vi "Periodic Tasks.vi"(8 "error in":errorcluster) -> ()   [LabVIEW 2015]
doc: "This VI runs in parallel to other tasks. It can contain as many user-defined periodic loops as you need. These can carry out PID or other sorts of timed response."
uses:
  <vilib>/Rock Robotics/WPI/CAN/TalonSRX/WPI_CANTalonSRX_APIControlMode.ctl
  Robot Global Data.vi
  <vilib>/Rock Robotics/WPI/Ultrasonic/WPI_SonarMB1010DigitalRefNum Registry Get.vi
  <vilib>/Rock Robotics/WPI/Ultrasonic/WPI_SonarMB1010DigitalGetRange.vi
  <vilib>/Rock Robotics/Network Tables/NT Write Number.vi
  <vilib>/Rock Robotics/Network Tables/NT Read Number.vi
  <vilib>/addons/control/pid/pid.llb/PID (DBL).vi
  navx-mxp/labview/navX Library v2/navX Library v2.lvlib
  <vilib>/addons/control/pid/NI_PID_pid.lvlib
panel:
  out "Motor Output 2":dbl(graph)
  in  "Intake delay":u32
  in  "Accuracy (+/-)":dbl=0.001 format="%#_13g"
  out "Sensor Velocity":dbl
  out "Distance 2":dbl
  in  "Ramp Rate 2":dbl
  in  "P 2":dbl=0.04
  in  "I 2":dbl=0.000122
  in  "D 2":dbl=0.7
  in  "F 2":dbl=0.0096
  in  "I Zone 2":dbl
  in  "Post beam break delay":u32=200
  in  "Ramp Rate":dbl
  in  "I Zone":dbl
  in  "F":dbl=0.0088
  in  "D":dbl
  in  "I":dbl
  in  "P":dbl
  in  "PID gains Lvl 3":T1={"proportional gain (Kc)"=2.0, "integral time (Ti, min)"=0.0, "derivative time (Td, min)"=0.0003}
  out "Pitch":dbl
  in  "PID Gains Lvl 1":T1={"proportional gain (Kc)"=3.0, "integral time (Ti, min)"=0.0, "derivative time (Td, min)"=0.0}
  out "Motor Output":dbl(graph)
  in  "PID Gains lv 2":T1={"proportional gain (Kc)"=9.0, "integral time (Ti, min)"=0.0, "derivative time (Td, min)"=0.0003}
  out "Potentiometer":dbl
  out "Beam Brake Tripped?":bool
  out "Yaw":dbl
  out "Roll":dbl
  in  "Command limit":dbl=0.25
  in  "Yaw Reset":bool
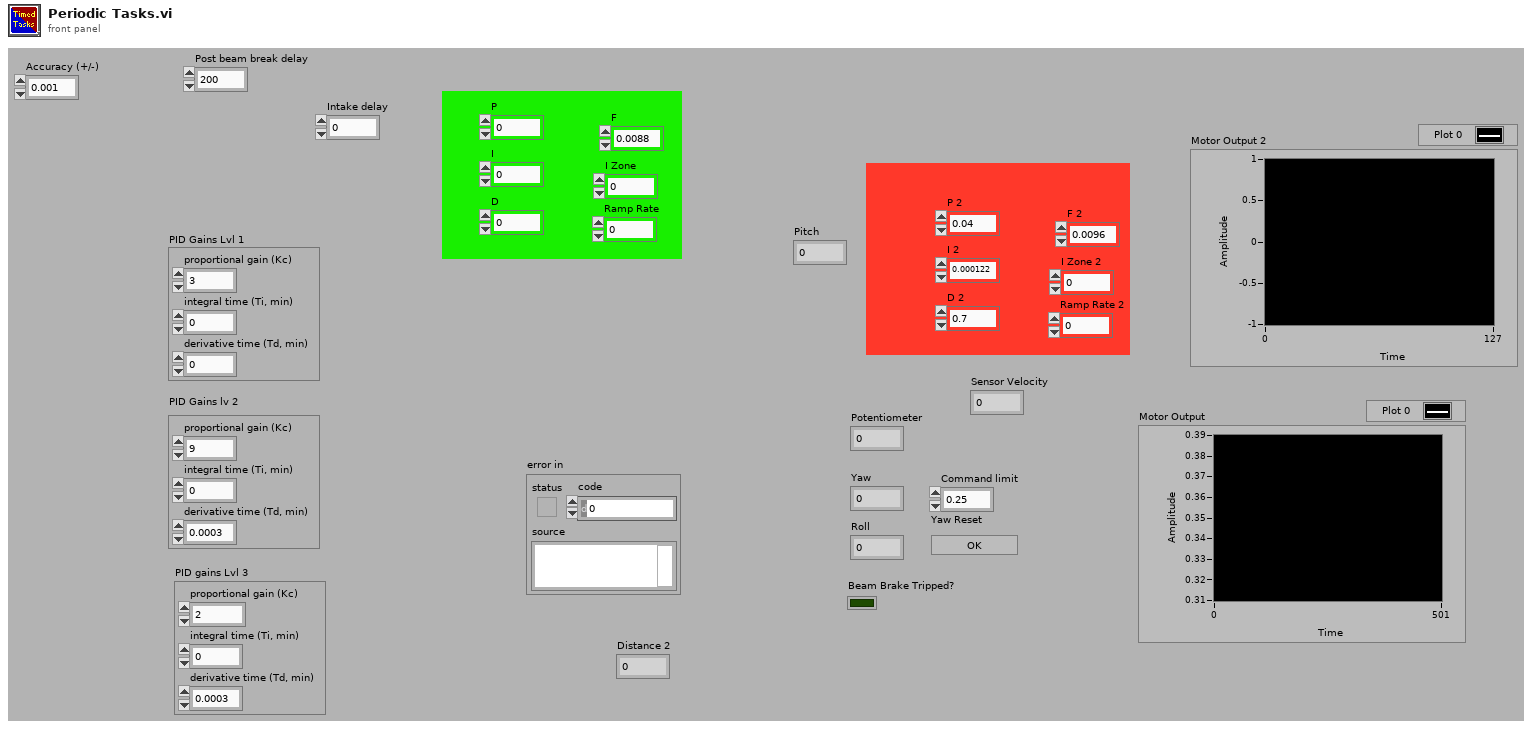
[diagram p1: front panel]
types:
  T1 = cluster{"proportional gain (Kc)":dbl, "integral time (Ti, min)":dbl, "derivative time (Td, min)":dbl}
  T2 = typedef "WPI_SonarMB1010DigitalDeviceRef.ctl" = cluster{"CounterDevRef":T3, "Scaling factor (s/in)":dbl}
  T3 = typedef "WPI_CounterDevRef.ctl" = cluster{"DevStatus":errorcluster, "CntIndex":T4}
  T4 = typedef "FPGA_CounterCtrSystemIndex.ctl" = enum8{"Ctr 0", "Ctr 1", "Ctr 2", "Ctr 3", "Ctr 4", "Ctr 5", "Ctr 6", "Ctr 7", "Invalid"}
  T5 = typedef "navX Library v2.lvlib/Z900_navX_DeviceTypeDef.ctl" = cluster{"Interface":cluster{"Protocol":T6, "Update Rate (4Hz-60Hz)":u8, "navX Open TypeDef":variant}, "Notify Packet":refnum<notifier>, "Loop VI Refnum":refnum<vi>, "Ready to Close Occurrence Refnum":refnum<k4>}
  T6 = typedef "navX Library v2.lvlib/Z900_navX_ProtocolTypeDef.ctl" = enum16{"SERIAL", "I2C", "SPI"}
  T7 = typedef "WPI_PotentiometerDevRef.ctl" = cluster{"DevStatus":errorcluster, "Analog Channel":T8, "Invert Output":bool}
  T8 = typedef "FPGA_AIChannel.ctl" = enum8{"AI 0", "AI 1", "AI 2", "AI 3", "AI MXP 0", "AI MXP 1", "AI MXP 2", "AI MXP 3", "Invalid"}
  T9 = cluster{"Yaw":dbl, "Roll":dbl, "Pitch":dbl, "Heading":dbl, "Fused Heading":dbl}
  T10 = typedef "WPI_DigitalInputDevRef.ctl" = cluster{"DevStatus":errorcluster, "DIO Channel":T11}
  T11 = typedef "FPGA_DIOChannel.ctl" = enum8{"DIO 0", "DIO 1", "DIO 2", "DIO 3", "DIO 4", "DIO 5", "DIO 6", "DIO 7", "DIO 8", "DIO 9", "DIO MXP 0", "DIO MXP 1", "DIO MXP 2", "DIO MXP 3", "DIO MXP 4", "DIO MXP 5", "DIO MXP 6", "DIO MXP 7", "DIO MXP 8", "DIO MXP 9", "DIO MXP 10", "DIO MXP 11", "DIO MXP 12", "DIO MXP 13", "DIO MXP 14", "DIO MXP 15", "Invalid"}
  T12 = typedef "WPI_MotorControlDeviceRef.ctl" = cluster{"DeviceStatus":errorcluster, "Type":T13, "PWM":cluster{"PWM Channel":T14, "DeadBand":T15}, "CAN":cluster{"Device Number":u8, "Control Mode":T16, "Semaphore":T17, "Max Vout":dbl, "TalonSRX Control Mode":T18}, "Invert":bool}
  T13 = typedef "WPI_MotorControlType.ctl" = enum16{"PWM", "CAN", "CANTalonSRX"}
  T14 = typedef "FPGA_DIOPWMChannel.ctl" = enum8{"PWM 0", "PWM 1", "PWM 2", "PWM 3", "PWM 4", "PWM 5", "PWM 6", "PWM 7", "PWM 8", "PWM 9", "PWM MXP 0", "PWM MXP 1", "PWM MXP 2", "PWM MXP 3", "PWM MXP 4", "PWM MXP 5", "PWM MXP 6", "PWM MXP 7", "PWM MXP 8", "PWM MXP 9", "Invalid"}
  T15 = typedef "WPI_PWMDeadband.ctl" = cluster{"Name":string, "maxPositivePwm":i32, "minPositivePwm":i32, "centerPwm":i32, "maxNegativePwm":i32, "minNegativePwm":i32, "angularRange":u16}
  T16 = typedef "WPI_CANJaguar_ControlMode.ctl" = enum8{"Percent VBus", "Current", "Speed", "Position", "Voltage"}
  T17 = typedef "Semaphore RefNum" = refnum<k1>
  T18 = typedef "WPI_CANTalonSRX_APIControlMode.ctl" = enum8{"Percent VBus", "Speed", "Position", "Slave", "Unchanged / Invalid", "Voltage Compensation", "Current", "Motion Profile"}
  T19 = typedef "WPI_CANTalonSRX_GlobalStatus.ctl" = cluster{"Applied Throttle":dbl, "Module Enabled":bool, "CAN Error":errorcluster, "Closed Loop Error":dbl, "Forward Limit Switch Closed":bool, "Reverse Limit Switch Closed":bool, "Sensor Position":dbl, "Sensor Velocity":dbl, "Current":dbl, "Sticky Fault - Over Temp":bool, "Sticky Fault - Under Voltage":bool, "Sticky Fault - Forward Limit":bool, "Sticky Fault - Reverse Limit":bool, "Sticky Fault - Forward Soft Limit":bool, "Sticky Fault - Reverse Soft Limit":bool, "Brake is Enabled":bool, "Encoder Position":dbl, "Encoder Velocity":dbl, "Encoder Index Count":dbl, "Encoder A Pin State":bool, "Encoder B Pin State":bool, "Encoder Index Pin State":bool, "Analog In":dbl, "Analog In Velocity":dbl, "Temperature (C)":dbl, "Battery Voltage":dbl, "Control 5 Is Supported":bool, "Current Profile Slot Select":dbl, "Pos Div 8":bool, "Vel Div 4":bool, "Pulse Width Position":i32, "Pulse Width Velocity":i32, "Pulse Width Rise To Rise (us)":i32, "Pulse Width Rise To Fall (us)":i32, "Mot Prof Active Is Under Run":bool, "Mot Prof Active Has Under Run":bool, "Mot Prof Active Is Last":bool, "Mot Prof Active Velocity Only":bool, "Mot Prof Active Is Valid":bool, "Mot Prof Buffer Is Full":bool, "Mot Prof Active Profile Slot Select":i32, "Mot Prof NextID":i32, "Mot Prof Count":i32, "Mot Prof Active Velocity":dbl, "Mot Prof Active Position":dbl, "Mot Prof Output Enable":i32}
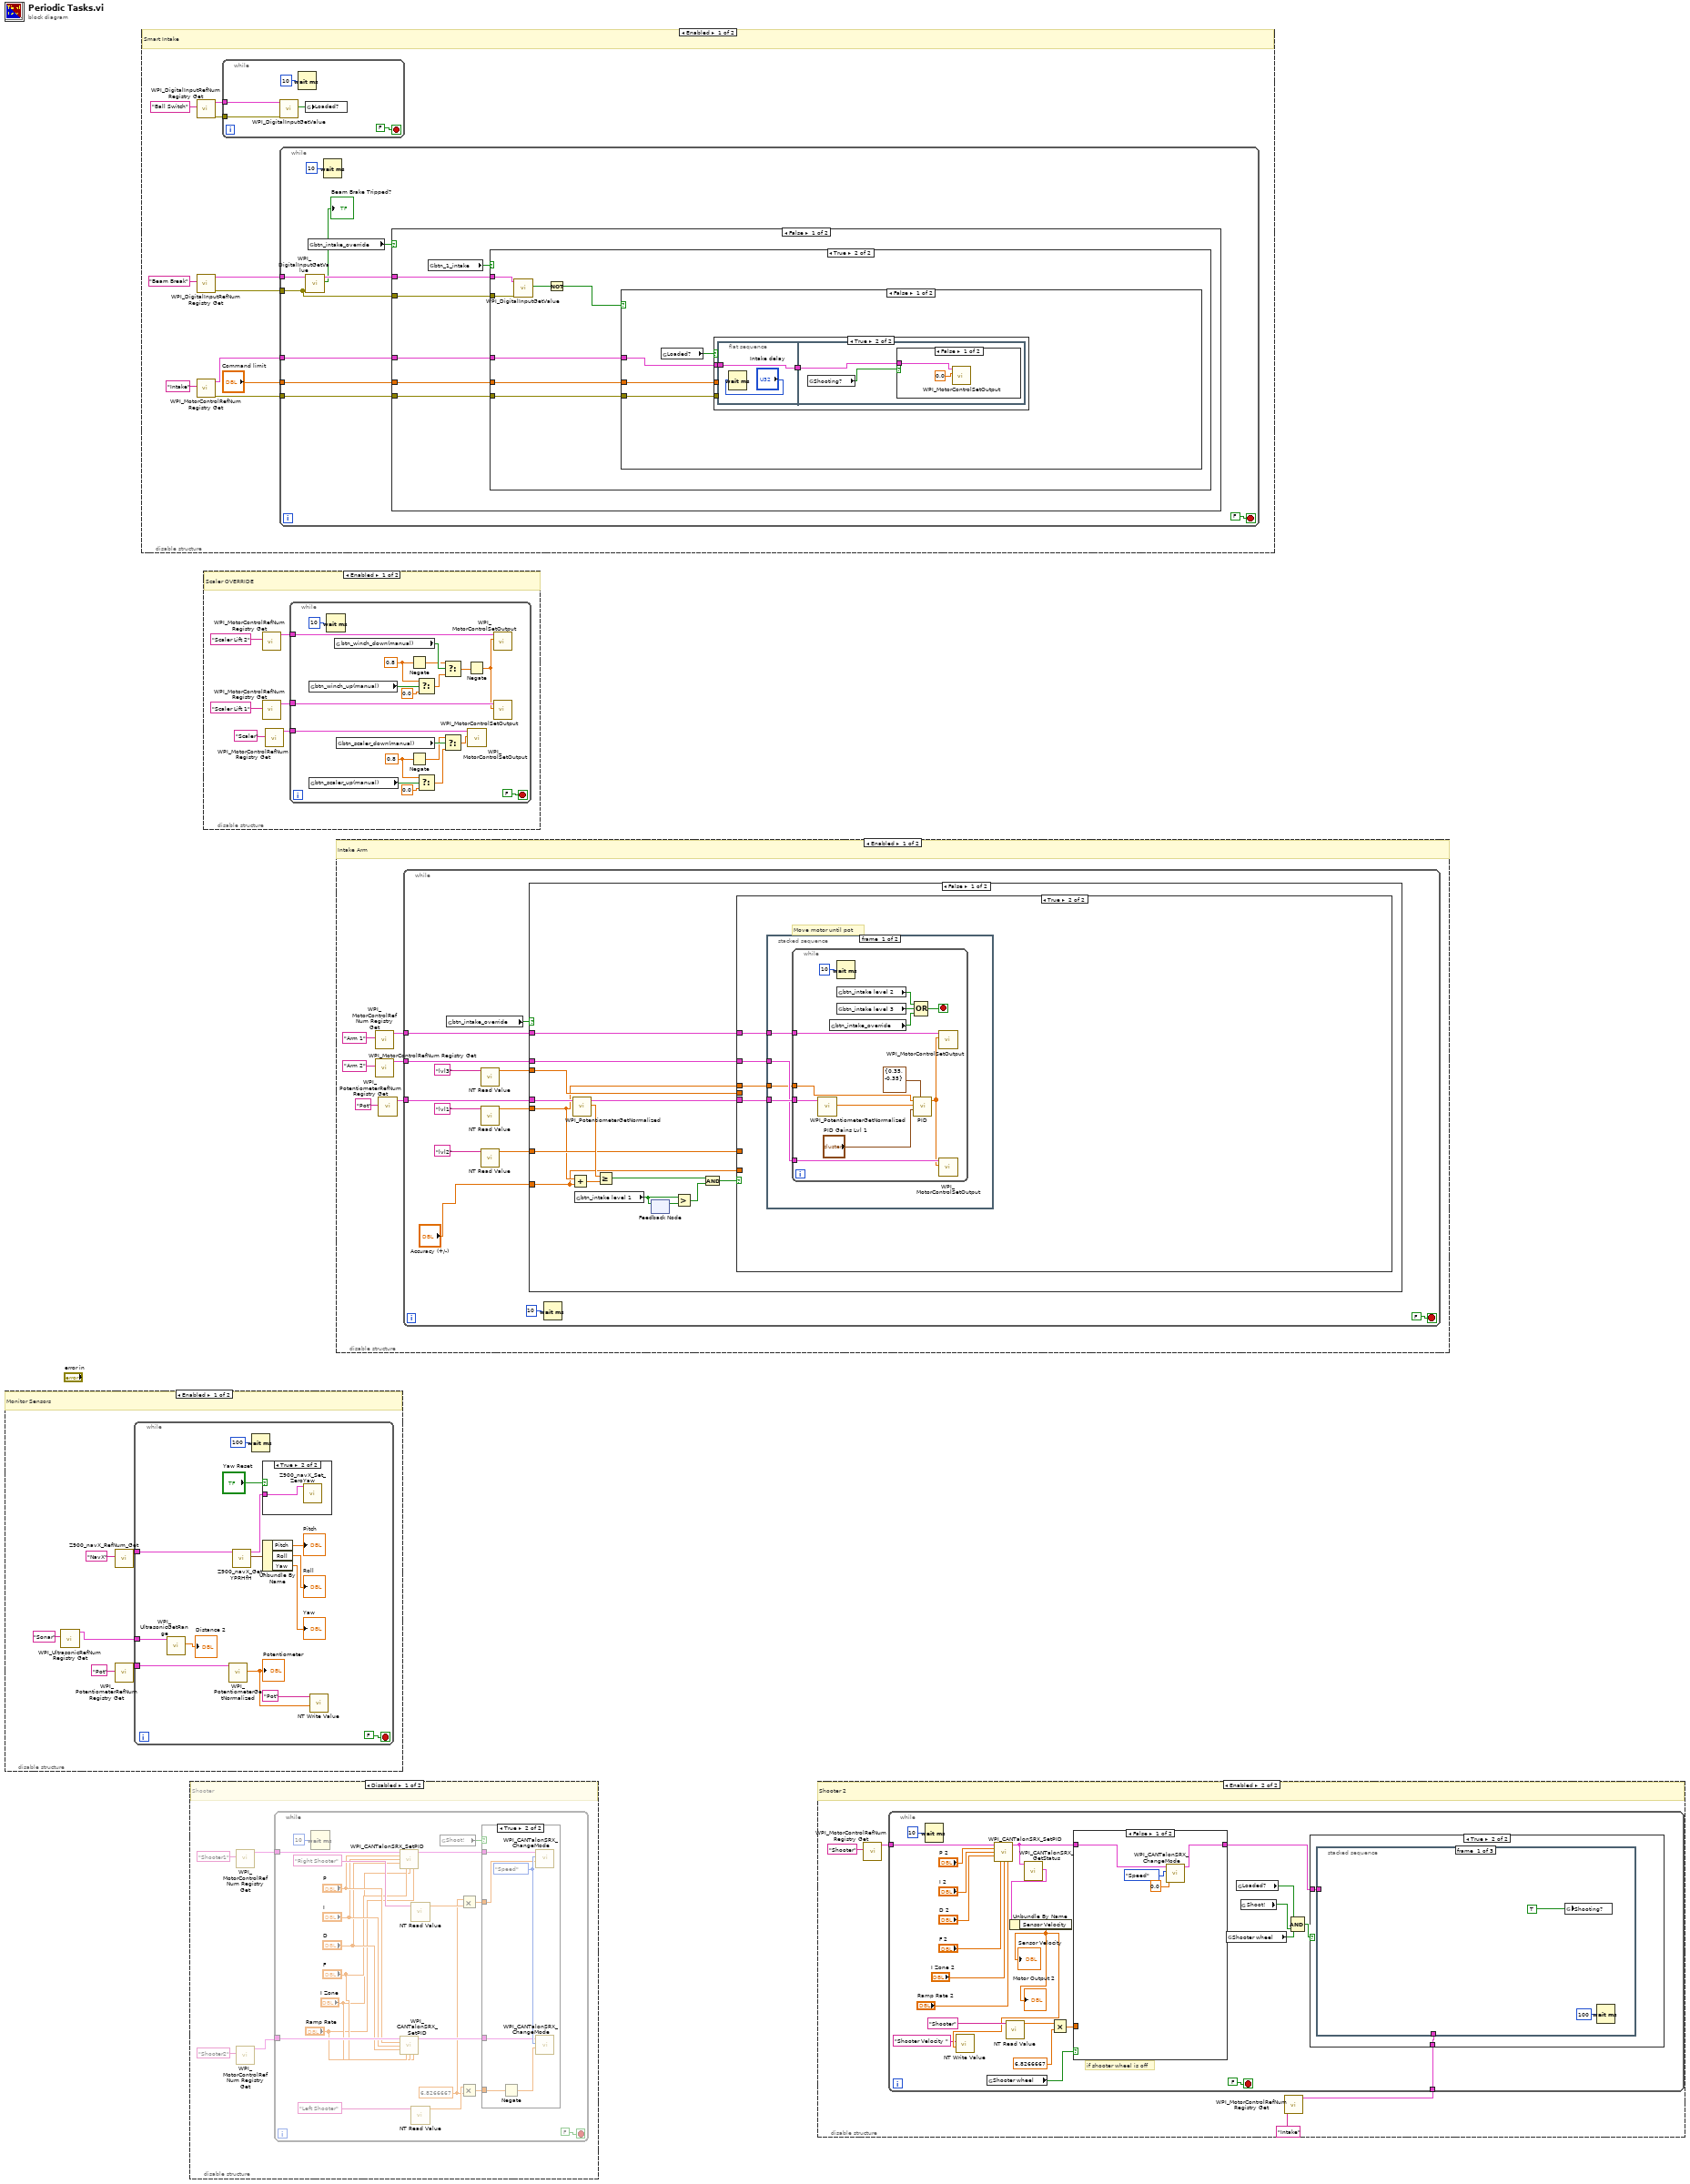
[diagram p0: block diagram]
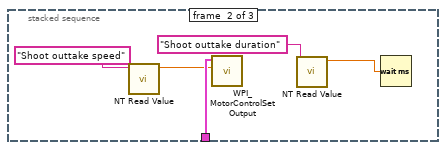
[diagram p4: hidden frame]
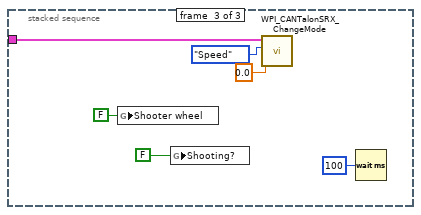
[diagram p5: hidden frame]
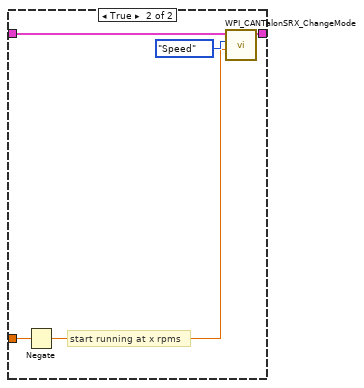
[diagram p6: hidden frame]
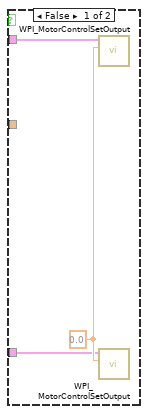
[diagram p7: hidden frame]
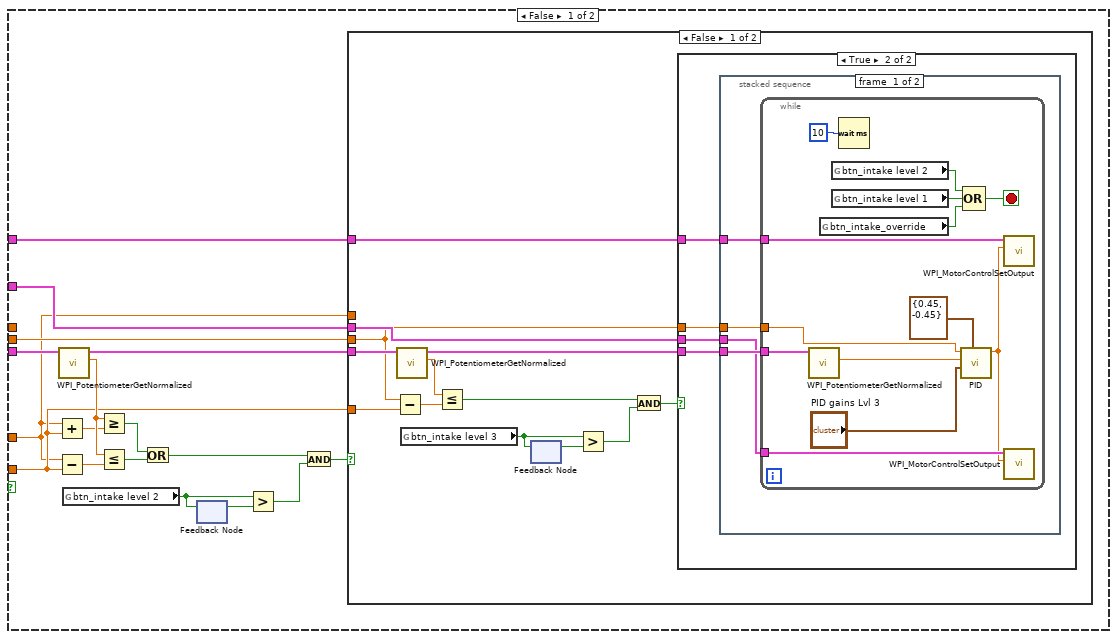
[diagram p10: hidden frame]
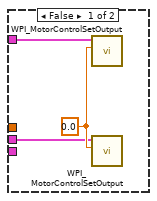
[diagram p11: hidden frame]
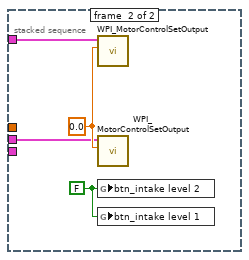
[diagram p12: hidden frame]
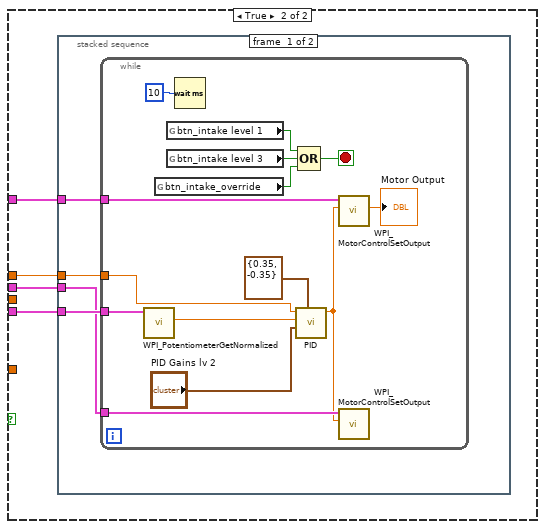
[diagram p13: hidden frame]
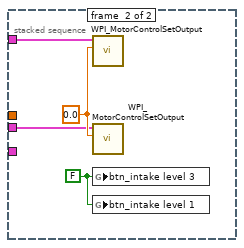
[diagram p14: hidden frame]
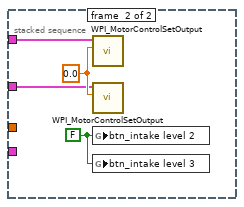
[diagram p15: hidden frame]
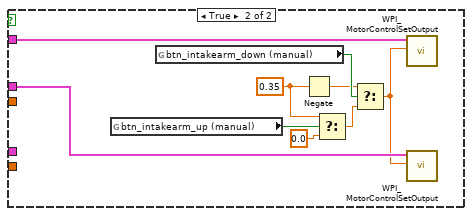
[diagram p16: hidden frame]
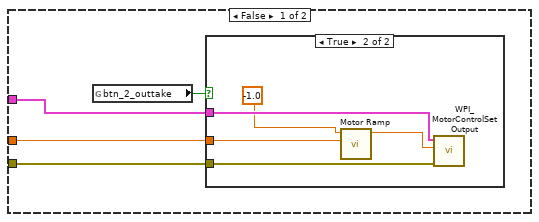
[diagram p20: hidden frame]
diagram:
  n1 = disable-structure shown="Enabled" {
    frame Enabled {
      # "Monitor Sensors"
      n2 = call-poly <vilib>:"WPI_UltrasonicRefNum Registry Get.vi"("refnum name"="Sonar") -> ("SonarMB1010DigitalDevRef"=w1:T2)  [unwired: 9 in, 1 out]
      n3 = call "Z900_navX_RefNum_Get.vi"("refnum name"="NavX") -> ("navX Device"=w5:T5)  [unwired: 9 in, 1 out]
      n4 = call <vilib>:"WPI_PotentiometerRefNum Registry Get.vi"("refnum name"="Pot") -> ("PotDevRef"=w3:T7)  [unwired: 9 in, 1 out]
      n5 = while {
        tunnel: w5 -> [w16]
        tunnel: w3 -> [w12]
        tunnel: w1 -> [w8]
        stop <- FALSE stop-if-true
        # "NavX Status"
        n6 = call-poly <vilib>:"WPI_UltrasonicGetRange.vi"("SonarMB1010DigitalDevRef"=w8) -> ("Distance"=→"Distance 2":dbl)  [unwired: 8 in, 2 out]
        n7 = call <vilib>:"WPI_PotentiometerGetNormalized.vi"("PotDevRef"=w12) -> ("Normalized Value"=w10:dbl)  [unwired: 8 in, 2 out]
        "Potentiometer" <- w10
        n8 = call "Z900_navX_Get_YPRHfH.vi"("navX Device"=w16) -> ("YRPHfH"=w13:T9, "navX Device"=w15:T5)  [unwired: 7 in, 2 out]
        n9 = Wait (ms)(milliseconds to wait=u32 100) -> ()  [unwired: 1 out]
        n10 = case shown="True" "Yaw Reset" {
          tunnel: w15 -> [_ w21]
          frame False {
          }
          frame True {
            n11 = call "Z900_navX_Set_ZeroYaw.vi"("navX Device"=w21) -> ()  [unwired: 9 in, 2 out]
          }
        }
        n12 = Unbundle By Name(w13) -> ("Pitch"=→"Pitch":dbl, "Roll"=→"Roll":dbl, "Yaw"=→"Yaw":dbl)
        n13 = call-poly <vilib>:"NT Write Value.vi"("Numeric"=w10, "Name"="Pot") -> ()  [unwired: 9 in, 1 out]
      }
    }
    frame Disabled {
    }
  }
  n14 = disable-structure shown="Enabled" {
    frame Enabled {
      # "Smart Intake"
      n15 = call <vilib>:"WPI_DigitalInputRefNum Registry Get.vi"("refnum name"="Ball Switch") -> ("error out"=w23:errorcluster, "DigitalInputDevRef"=w22:T10)  [unwired: 9 in]
      n16 = call <vilib>:"WPI_DigitalInputRefNum Registry Get.vi"("refnum name"="Beam Break") -> ("error out"=w31:errorcluster, "DigitalInputDevRef"=w30:T10)  [unwired: 9 in]
      n17 = call <vilib>:"WPI_MotorControlRefNum Registry Get.vi"("refnum name"="Intake") -> ("error out"=w28:errorcluster, "MotorControlDevRef"=w27:T12)  [unwired: 9 in]
      n18 = while {
        tunnel: w23 -> [w36]
        tunnel: w22 -> [w35]
        stop <- FALSE stop-if-true
        n19 = call <vilib>:"WPI_DigitalInputGetValue.vi"("error in (no error)"=w36, "DigitalInputDevRef"=w35) -> ("Value"=w32:bool)  [unwired: 7 in, 2 out]
        n20 = Wait (ms)(milliseconds to wait=u32 10) -> ()  [unwired: 1 out]
        n21 = global write "Robot Global Data.vi" "Loaded?"(w32) -> ()
      }
      n22 = while {
        tunnel: w30 -> [w46]
        tunnel: w31 -> [w39]
        tunnel: w27 -> [w45]
        tunnel: w28 -> [w44]
        tunnel: "Command limit" -> [w43]
        stop <- FALSE stop-if-true
        n23 = call <vilib>:"WPI_DigitalInputGetValue.vi"("error in (no error)"=w39, "DigitalInputDevRef"=w46) -> ("Value"=→"Beam Brake Tripped?":bool, "DigitalInputDevRef"=w40:T10)  [unwired: 7 in, 1 out]
        n24 = global read "Robot Global Data.vi" "btn_intake_override"() -> (w37:bool)
        n25 = Wait (ms)(milliseconds to wait=u32 10) -> ()  [unwired: 1 out]
        n26 = case shown="False" w37 {
          tunnel: w45 -> [w52 w119]
          tunnel: w44 -> [w51 _]
          tunnel: w43 -> [w50 _]
          tunnel: w40 -> [w48 _]
          tunnel: w39 -> [w47 _]
          frame False {
            n27 = global read "Robot Global Data.vi" "btn_1_intake"() -> (w49:bool)
            n28 = case shown="True" w49 {
              tunnel: w48 -> [_ w77]
              tunnel: w47 -> [_ w76]
              tunnel: w52 -> [w56 w75]
              tunnel: w51 -> [w55 w74]
              tunnel: w50 -> [w54 w73]
              frame False {
                n29 = global read "Robot Global Data.vi" "btn_2_outtake"() -> (w53:bool)
                n30 = case shown="True" w53 {
                  tunnel: w54 -> [w60 w70]
                  tunnel: w56 -> [w59 w69]
                  tunnel: w55 -> [w58 w68]
                  frame False {
                    n31 = global read "Robot Global Data.vi" "Shooting?"() -> (w57:bool)
                    n32 = case shown="False" w57 {
                      tunnel: w60 -> [w65 _]
                      tunnel: w59 -> [w64 _]
                      tunnel: w58 -> [w63 _]
                      frame False {
                        n33 = call "Motor Ramp.vi"("Command limit"=w65, "Joystick in"=0.0) -> ("Joystick out"=w62:dbl)  [unwired: 9 in]
                        n34 = call <vilib>:"WPI_MotorControlSetOutput.vi"("error in (no error)"=w63, "Output"=w62, "MotorControlDevRef"=w64) -> ()  [unwired: 6 in, 3 out]
                      }
                      frame True {
                      }
                    }
                  }
                  frame True {
                    n35 = call "Motor Ramp.vi"("Command limit"=w70, "Joystick in"=-1.0) -> ("Joystick out"=w67:dbl)  [unwired: 9 in]
                    n36 = call <vilib>:"WPI_MotorControlSetOutput.vi"("error in (no error)"=w68, "Output"=w67, "MotorControlDevRef"=w69) -> ()  [unwired: 6 in, 3 out]
                  }
                }
              }
              frame True {
                n37 = call <vilib>:"WPI_DigitalInputGetValue.vi"("error in (no error)"=w76, "DigitalInputDevRef"=w77) -> ("Value"=w71:bool)  [unwired: 7 in, 2 out]
                n38 = Not(x=w71) -> (.not. x?=w72:bool)
                n39 = case shown="False" w72 {
                  tunnel: w75 -> [w81 w99]
                  tunnel: w74 -> [w80 w98]
                  tunnel: w73 -> [w79 w97]
                  frame False {
                    n40 = global read "Robot Global Data.vi" "Loaded?"() -> (w78:bool)
                    n41 = case shown="True" w78 {
                      tunnel: w79 -> [w84 _]
                      tunnel: w81 -> [w86 w88]
                      tunnel: w80 -> [w83 _]
                      frame False {
                        n42 = call "Motor Ramp.vi"("Command limit"=w84, "Joystick in"=0.8 ("Slow intake")) -> ("Joystick out"=w85:dbl)  [unwired: 9 in]
                        n43 = call <vilib>:"WPI_MotorControlSetOutput.vi"("error in (no error)"=w83, "Output"=w85, "MotorControlDevRef"=w86) -> ()  [unwired: 6 in, 3 out]
                      }
                      frame True {
                        n44 = flat-sequence {
                          tunnel: w88 -> [w90]
                          tunnel: [w90] -> w87
                          tunnel: w87 -> [w91]
                          frame #0 {
                            n45 = Wait (ms)(milliseconds to wait="Intake delay") -> ()  [unwired: 1 out]
                          }
                          frame #1 {
                            n46 = global read "Robot Global Data.vi" "Shooting?"() -> (w92:bool)
                            n47 = case shown="False" w92 {
                              tunnel: w91 -> [w94 _]
                              frame False {
                                n48 = call <vilib>:"WPI_MotorControlSetOutput.vi"("Output"=0.0, "MotorControlDevRef"=w94) -> ()  [unwired: 7 in, 3 out]
                              }
                              frame True {
                              }
                            }
                          }
                        }
                      }
                    }
                  }
                  frame True {
                    n49 = flat-sequence {
                      tunnel: w99 -> [w103]
                      tunnel: w98 -> [w102]
                      tunnel: w97 -> [w101]
                      tunnel: [w100] -> w96
                      tunnel: w96 -> [w113]
                      tunnel: [w113] -> w95
                      tunnel: w95 -> [w115]
                      frame #0 {
                        n50 = while {
                          tunnel: w103 -> [w111]
                          tunnel: w102 -> [w110]
                          tunnel: w101 -> [w109]
                          tunnel: [w105] -> w100
                          stop <- w106 stop-if-true
                          n51 = Wait (ms)(milliseconds to wait=u32 10) -> ()  [unwired: 1 out]
                          n52 = call "Motor Ramp.vi"("Command limit"=w109, "Joystick in"=0.6 ("Fast intake")) -> ("Joystick out"=w108:dbl)  [unwired: 9 in]
                          n53 = global read "Robot Global Data.vi" "Loaded?"() -> (w106:bool)
                          n54 = call <vilib>:"WPI_MotorControlSetOutput.vi"("error in (no error)"=w110, "Output"=w108, "MotorControlDevRef"=w111) -> ("MotorControlDevRef"=w105:T12)  [unwired: 6 in, 2 out]
                        }
                      }
                      frame #1 {
                        n55 = Wait (ms)(milliseconds to wait="Post beam break delay") -> ()  [unwired: 1 out]
                      }
                      frame #2 {
                        n56 = global read "Robot Global Data.vi" "Shooting?"() -> (w114:bool)
                        n57 = case shown="False" w114 {
                          tunnel: w115 -> [w116 _]
                          frame False {
                            n58 = call <vilib>:"WPI_MotorControlSetOutput.vi"("Output"=0.0, "MotorControlDevRef"=w116) -> ()  [unwired: 7 in, 3 out]
                          }
                          frame True {
                          }
                        }
                      }
                    }
                  }
                }
              }
            }
          }
          frame True {
            n59 = global read "Robot Global Data.vi" "btn_2_outtake"() -> (w122:bool)
            n60 = global read "Robot Global Data.vi" "btn_1_intake"() -> (w125:bool)
            n61 = Select(t=-0.8, s=w122, f=0.0) -> (s? t:f=w123:dbl)
            n62 = Select(t=0.6, s=w125, f=w123) -> (s? t:f=w118:dbl)
            n63 = call <vilib>:"WPI_MotorControlSetOutput.vi"("Output"=w118, "MotorControlDevRef"=w119) -> ()  [unwired: 7 in, 3 out]
          }
        }
      }
    }
    frame Disabled {
    }
  }
  n64 = disable-structure shown="Disabled" {
    frame Disabled {
      # "Shooter"
      n65 = call <vilib>:"WPI_MotorControlRefNum Registry Get.vi"("refnum name"="Shooter1") -> ("MotorControlDevRef"=w127:T12)  [unwired: 9 in, 1 out]
      n66 = call <vilib>:"WPI_MotorControlRefNum Registry Get.vi"("refnum name"="Shooter2") -> ("MotorControlDevRef"=w126:T12)  [unwired: 9 in, 1 out]
      n67 = while {
        tunnel: w127 -> [w149]
        tunnel: w126 -> [w148]
        stop <- FALSE stop-if-true
        w136 = 6.8266667 ("y")
        n68 = Wait (ms)(milliseconds to wait=u32 10) -> ()  [unwired: 1 out]
        n69 = call <vilib>:"WPI_CANTalonSRX_SetPID.vi"("CAN Talon SRX Ref"=w149, "P"="P", "I"="I", "D"="D", "F"="F", "I Zone"="I Zone", "Ramp Rate"="Ramp Rate") -> ("CAN Talon SRX Ref"=w144:T12)  [unwired: 7 in, 1 out]
        n70 = call <vilib>:"WPI_CANTalonSRX_SetPID.vi"("CAN Talon SRX Ref"=w148, "P"="P", "I"="I", "D"="D", "F"="F", "I Zone"="I Zone", "Ramp Rate"="Ramp Rate") -> ("CAN Talon SRX Ref"=w145:T12)  [unwired: 7 in, 1 out]
        n71 = call-poly <vilib>:"NT Read Value.vi"("Name"="Right Shooter") -> ("Numeric"=w142:dbl)  [unwired: 9 in, 1 out]
        n72 = call-poly <vilib>:"NT Read Value.vi"("Name"="Left Shooter") -> ("Numeric"=w143:dbl)  [unwired: 9 in, 1 out]
        n73 = global read "Robot Global Data.vi" "Shoot!"() -> (w139:bool)
        n74 = Multiply(x=w136, y=w142) -> (x*y=w137:dbl)
        n75 = Multiply(x=w143, y=w136) -> (x*y=w138:dbl)
        n76 = case shown="True" w139 {
          tunnel: w145 -> [w151 w157]
          tunnel: w144 -> [w150 w156]
          tunnel: w138 -> [_ w155]
          tunnel: w137 -> [_ w154]
          frame False {
            w152 = 0.0 ("Output")
            n77 = call <vilib>:"WPI_MotorControlSetOutput.vi"("Output"=w152, "MotorControlDevRef"=w150) -> ()  [unwired: 7 in, 3 out]
            n78 = call <vilib>:"WPI_MotorControlSetOutput.vi"("Output"=w152, "MotorControlDevRef"=w151) -> ()  [unwired: 7 in, 3 out]
          }
          frame True {
            w158 = WPI_CANTalonSRX_APIControlMode."Speed" ("Control Mode")
            n79 = Negate(x=w155) -> (-x=w153:dbl)
            n80 = call <vilib>:"WPI_CANTalonSRX_ChangeMode.vi"("Output"=w154, "Control Mode"=w158, "CAN Talon SRX Ref"=w156) -> ()  [unwired: 7 in, 2 out]
            n81 = call <vilib>:"WPI_CANTalonSRX_ChangeMode.vi"("Output"=w153, "Control Mode"=w158, "CAN Talon SRX Ref"=w157) -> ()  [unwired: 7 in, 2 out]
          }
        }
      }
    }
    frame Enabled {
    }
  }
  n82 = disable-structure shown="Enabled" {
    frame Enabled {
      # "Scaler OVERRIDE"
      n83 = call <vilib>:"WPI_MotorControlRefNum Registry Get.vi"("refnum name"="Scaler Lift 2") -> ("MotorControlDevRef"=w161:T12)  [unwired: 9 in, 1 out]
      n84 = call <vilib>:"WPI_MotorControlRefNum Registry Get.vi"("refnum name"="Scaler Lift 1") -> ("MotorControlDevRef"=w159:T12)  [unwired: 9 in, 1 out]
      n85 = call <vilib>:"WPI_MotorControlRefNum Registry Get.vi"("refnum name"="Scaler") -> ("MotorControlDevRef"=w162:T12)  [unwired: 9 in, 1 out]
      n86 = while {
        tunnel: w162 -> [w182]
        tunnel: w161 -> [w181]
        tunnel: w159 -> [w180]
        stop <- FALSE stop-if-true
        w168 = 0.8 ("t")
        w177 = 0.8 ("t")
        n87 = global read "Robot Global Data.vi" "btn_winch_up(manual)"() -> (w174:bool)
        n88 = global read "Robot Global Data.vi" "btn_scaler_up(manual)"() -> (w166:bool)
        n89 = Wait (ms)(milliseconds to wait=u32 10) -> ()  [unwired: 1 out]
        n90 = global read "Robot Global Data.vi" "btn_winch_down(manual)"() -> (w179:bool)
        n91 = global read "Robot Global Data.vi" "btn_scaler_down(manual)"() -> (w172:bool)
        n92 = Negate(x=w177) -> (-x=w176:dbl)
        n93 = Negate(x=w168) -> (-x=w169:dbl)
        n94 = Select(t=w177, s=w174, f=0.0) -> (s? t:f=w178:dbl)
        n95 = Select(t=w168, s=w166, f=0.0) -> (s? t:f=w171:dbl)
        n96 = Select(t=w176, s=w179, f=w178) -> (s? t:f=w173:dbl)
        n97 = Select(t=w169, s=w172, f=w171) -> (s? t:f=w167:dbl)
        n98 = Negate(x=w173) -> (-x=w165:dbl)
        n99 = call <vilib>:"WPI_MotorControlSetOutput.vi"("Output"=w167, "MotorControlDevRef"=w182) -> ()  [unwired: 7 in, 3 out]
        n100 = call <vilib>:"WPI_MotorControlSetOutput.vi"("Output"=w165, "MotorControlDevRef"=w181) -> ()  [unwired: 7 in, 3 out]
        n101 = call <vilib>:"WPI_MotorControlSetOutput.vi"("Output"=w165, "MotorControlDevRef"=w180) -> ()  [unwired: 7 in, 3 out]
      }
    }
    frame Disabled {
    }
  }
  n102 = disable-structure shown="Enabled" {
    frame Enabled {
      # "Intake Arm"
      n103 = call <vilib>:"WPI_MotorControlRefNum Registry Get.vi"("refnum name"="Arm 1") -> ("MotorControlDevRef"=w186:T12)  [unwired: 9 in, 1 out]
      n104 = call <vilib>:"WPI_MotorControlRefNum Registry Get.vi"("refnum name"="Arm 2") -> ("MotorControlDevRef"=w185:T12)  [unwired: 9 in, 1 out]
      n105 = call <vilib>:"WPI_PotentiometerRefNum Registry Get.vi"("refnum name"="Pot") -> ("PotDevRef"=w187:T7)  [unwired: 9 in, 1 out]
      n106 = while {
        tunnel: w187 -> [w202]
        tunnel: w186 -> [w201]
        tunnel: w185 -> [w200]
        stop <- FALSE stop-if-true
        n107 = global read "Robot Global Data.vi" "btn_intake_override"() -> (w198:bool)
        n108 = call-poly <vilib>:"NT Read Value.vi"("Name"="lvl3") -> ("Numeric"=w196:dbl)  [unwired: 9 in, 1 out]
        n109 = call-poly <vilib>:"NT Read Value.vi"("Name"="lvl1") -> ("Numeric"=w197:dbl)  [unwired: 9 in, 1 out]
        n110 = call-poly <vilib>:"NT Read Value.vi"("Name"="lvl2") -> ("Numeric"=w192:dbl)  [unwired: 9 in, 1 out]
        n111 = case shown="False" w198 {
          tunnel: w202 -> [w213 _]
          tunnel: w201 -> [w211 w336]
          tunnel: w200 -> [w210 w335]
          tunnel: w196 -> [w207 _]
          tunnel: w192 -> [w206 _]
          tunnel: w197 -> [w205 _]
          tunnel: "Accuracy (+/-)" -> [w204 _]
          frame False {
            n112 = Add(x=w205, y=w204) -> (x+y=w208:dbl)
            n113 = call <vilib>:"WPI_PotentiometerGetNormalized.vi"("PotDevRef"=w213) -> ("Normalized Value"=w209:dbl, "PotDevRef"=w212:T7)  [unwired: 8 in, 1 out]
            n114 = global read "Robot Global Data.vi" "btn_intake level 1"() -> (w214:bool)
            n115 = Greater Or Equal?(x=w209, y=w208) -> (x >= y?=w217:bool)
            n116 = feedback #1() -> (w215:bool)  [unwired: 1 in]
            n117 = feedback-in #1(w214) -> ()
            n118 = Greater?(x=w214, y=w215) -> (0:w216:bool)
            n119 = And(x=w217, y=w216) -> (x .and. y?=w218:bool)
            n120 = case shown="True" w218 {
              tunnel: w212 -> [w228 w306]
              tunnel: w211 -> [w225 w305]
              tunnel: w210 -> [w224 w304]
              tunnel: w204 -> [w221 _]
              tunnel: w207 -> [w220 _]
              tunnel: w206 -> [w219 _]
              tunnel: w205 -> [_ w303]
              frame False {
                n121 = Add(x=w219, y=w221) -> (x+y=w223:dbl)
                n122 = Subtract(x=w219, y=w221) -> (x-y=w222:dbl)
                n123 = call <vilib>:"WPI_PotentiometerGetNormalized.vi"("PotDevRef"=w228) -> ("Normalized Value"=w229:dbl, "PotDevRef"=w227:T7)  [unwired: 8 in, 1 out]
                n124 = global read "Robot Global Data.vi" "btn_intake level 2"() -> (w230:bool)
                n125 = Greater Or Equal?(x=w229, y=w223) -> (x >= y?=w226:bool)
                n126 = Less Or Equal?(x=w229, y=w222) -> (x <= y?=w234:bool)
                n127 = Or(x=w226, y=w234) -> (x .or. y?=w232:bool)
                n128 = feedback #2() -> (w235:bool)  [unwired: 1 in]
                n129 = feedback-in #2(w230) -> ()
                n130 = Greater?(x=w230, y=w235) -> (0:w233:bool)
                n131 = And(x=w232, y=w233) -> (x .and. y?=w231:bool)
                n132 = case shown="False" w231 {
                  tunnel: w227 -> [w242 w280]
                  tunnel: w225 -> [w239 w279]
                  tunnel: w224 -> [w240 w278]
                  tunnel: w221 -> [w237 _]
                  tunnel: w220 -> [w236 _]
                  tunnel: w219 -> [_ w277]
                  frame False {
                    n133 = Subtract(x=w236, y=w237) -> (x-y=w238:dbl)
                    n134 = call <vilib>:"WPI_PotentiometerGetNormalized.vi"("PotDevRef"=w242) -> ("Normalized Value"=w243:dbl, "PotDevRef"=w241:T7)  [unwired: 8 in, 1 out]
                    n135 = global read "Robot Global Data.vi" "btn_intake level 3"() -> (w244:bool)
                    n136 = Less Or Equal?(x=w243, y=w238) -> (x <= y?=w246:bool)
                    n137 = feedback #3() -> (w248:bool)  [unwired: 1 in]
                    n138 = feedback-in #3(w244) -> ()
                    n139 = Greater?(x=w244, y=w248) -> (0:w247:bool)
                    n140 = And(x=w246, y=w247) -> (x .and. y?=w245:bool)
                    n141 = case shown="True" w245 {
                      tunnel: w241 -> [_ w255]
                      tunnel: w240 -> [w249 w254]
                      tunnel: w239 -> [w250 w253]
                      tunnel: w236 -> [_ w252]
                      frame False {
                        w251 = 0.0 ("Output")
                        n142 = call <vilib>:"WPI_MotorControlSetOutput.vi"("Output"=w251, "MotorControlDevRef"=w250) -> ()  [unwired: 7 in, 3 out]
                        n143 = call <vilib>:"WPI_MotorControlSetOutput.vi"("Output"=w251, "MotorControlDevRef"=w249) -> ()  [unwired: 7 in, 3 out]
                      }
                      frame True {
                        n144 = stacked-sequence {
                          tunnel: w255 -> [w259 _]
                          tunnel: w254 -> [w258 w275]
                          tunnel: w253 -> [w257 w274]
                          tunnel: w252 -> [w256 _]
                          frame #0 {
                            n145 = while {
                              tunnel: w259 -> [w271]
                              tunnel: w258 -> [w270]
                              tunnel: w257 -> [w269]
                              tunnel: w256 -> [w261]
                              stop <- w262 stop-if-true
                              n146 = call <vilib>:"WPI_PotentiometerGetNormalized.vi"("PotDevRef"=w271) -> ("Normalized Value"=w265:dbl)  [unwired: 8 in, 2 out]
                              n147 = global read "Robot Global Data.vi" "btn_intake_override"() -> (w260:bool)
                              n148 = global read "Robot Global Data.vi" "btn_intake level 2"() -> (w264:bool)
                              n149 = global read "Robot Global Data.vi" "btn_intake level 1"() -> (w263:bool)
                              n150 = Wait (ms)(milliseconds to wait=u32 10) -> ()  [unwired: 1 out]
                              n151 = call-poly <vilib>:"PID.vi"("output range"=cluster{"output high":dbl, "output low":dbl} {"output high"=0.45, "output low"=-0.45}, "PID gains"="PID gains Lvl 3", "process variable"=w265, "setpoint"=w261) -> ("output"=w268:dbl)  [unwired: 6 in, 1 out]
                              n152 = Compound Arithmetic op=OR(w264, w263, w260) -> (w262:bool)
                              n153 = call <vilib>:"WPI_MotorControlSetOutput.vi"("Output"=w268, "MotorControlDevRef"=w269) -> ()  [unwired: 7 in, 3 out]
                              n154 = call <vilib>:"WPI_MotorControlSetOutput.vi"("Output"=w268, "MotorControlDevRef"=w270) -> ()  [unwired: 7 in, 3 out]
                            }
                          }
                          frame #1 {
                            w273 = FALSE ("btn_intake level 2")
                            w276 = 0.0 ("Output")
                            n155 = call <vilib>:"WPI_MotorControlSetOutput.vi"("Output"=w276, "MotorControlDevRef"=w274) -> ()  [unwired: 7 in, 3 out]
                            n156 = call <vilib>:"WPI_MotorControlSetOutput.vi"("Output"=w276, "MotorControlDevRef"=w275) -> ()  [unwired: 7 in, 3 out]
                            n157 = global write "Robot Global Data.vi" "btn_intake level 2"(w273) -> ()
                            n158 = global write "Robot Global Data.vi" "btn_intake level 1"(w273) -> ()
                          }
                        }
                      }
                    }
                  }
                  frame True {
                    n159 = stacked-sequence {
                      tunnel: w280 -> [w284 _]
                      tunnel: w279 -> [w283 w300]
                      tunnel: w278 -> [w282 w301]
                      tunnel: w277 -> [w281 _]
                      frame #0 {
                        n160 = while {
                          tunnel: w284 -> [w297]
                          tunnel: w283 -> [w296]
                          tunnel: w282 -> [w295]
                          tunnel: w281 -> [w285]
                          stop <- w288 stop-if-true
                          n161 = call <vilib>:"WPI_PotentiometerGetNormalized.vi"("PotDevRef"=w297) -> ("Normalized Value"=w291:dbl)  [unwired: 8 in, 2 out]
                          n162 = global read "Robot Global Data.vi" "btn_intake_override"() -> (w286:bool)
                          n163 = global read "Robot Global Data.vi" "btn_intake level 1"() -> (w290:bool)
                          n164 = global read "Robot Global Data.vi" "btn_intake level 3"() -> (w289:bool)
                          n165 = Wait (ms)(milliseconds to wait=u32 10) -> ()  [unwired: 1 out]
                          n166 = call-poly <vilib>:"PID.vi"("output range"=cluster{"output high":dbl, "output low":dbl} {"output high"=0.35, "output low"=-0.35}, "PID gains"="PID Gains lv 2", "process variable"=w291, "setpoint"=w285) -> ("output"=w292:dbl)  [unwired: 6 in, 1 out]
                          n167 = Compound Arithmetic op=OR(w290, w289, w286) -> (w288:bool)
                          n168 = call <vilib>:"WPI_MotorControlSetOutput.vi"("Output"=w292, "MotorControlDevRef"=w296) -> ("Motor Output"=→"Motor Output":dbl)  [unwired: 7 in, 2 out]
                          n169 = call <vilib>:"WPI_MotorControlSetOutput.vi"("Output"=w292, "MotorControlDevRef"=w295) -> ()  [unwired: 7 in, 3 out]
                        }
                      }
                      frame #1 {
                        w299 = FALSE ("btn_intake level 2")
                        w302 = 0.0 ("Output")
                        n170 = call <vilib>:"WPI_MotorControlSetOutput.vi"("Output"=w302, "MotorControlDevRef"=w300) -> ()  [unwired: 7 in, 3 out]
                        n171 = call <vilib>:"WPI_MotorControlSetOutput.vi"("Output"=w302, "MotorControlDevRef"=w301) -> ()  [unwired: 7 in, 3 out]
                        n172 = global write "Robot Global Data.vi" "btn_intake level 3"(w299) -> ()
                        n173 = global write "Robot Global Data.vi" "btn_intake level 1"(w299) -> ()
                      }
                    }
                  }
                }
              }
              frame True {
                # "Move motor until pot"
                n174 = stacked-sequence {
                  tunnel: w306 -> [w310 _]
                  tunnel: w305 -> [w309 w326]
                  tunnel: w304 -> [w308 w325]
                  tunnel: w303 -> [w307 _]
                  frame #0 {
                    n175 = while {
                      tunnel: w310 -> [w322]
                      tunnel: w309 -> [w321]
                      tunnel: w308 -> [w320]
                      tunnel: w307 -> [w312]
                      stop <- w313 stop-if-true
                      n176 = call <vilib>:"WPI_PotentiometerGetNormalized.vi"("PotDevRef"=w322) -> ("Normalized Value"=w314:dbl)  [unwired: 8 in, 2 out]
                      n177 = global read "Robot Global Data.vi" "btn_intake_override"() -> (w311:bool)
                      n178 = Wait (ms)(milliseconds to wait=u32 10) -> ()  [unwired: 1 out]
                      n179 = global read "Robot Global Data.vi" "btn_intake level 2"() -> (w317:bool)
                      n180 = global read "Robot Global Data.vi" "btn_intake level 3"() -> (w316:bool)
                      n181 = call-poly <vilib>:"PID.vi"("output range"=cluster{"output high":dbl, "output low":dbl} {"output high"=0.35, "output low"=-0.35}, "PID gains"="PID Gains Lvl 1", "process variable"=w314, "setpoint"=w312) -> ("output"=w315:dbl)  [unwired: 6 in, 1 out]
                      n182 = Compound Arithmetic op=OR(w317, w316, w311) -> (w313:bool)
                      n183 = call <vilib>:"WPI_MotorControlSetOutput.vi"("Output"=w315, "MotorControlDevRef"=w321) -> ()  [unwired: 7 in, 3 out]
                      n184 = call <vilib>:"WPI_MotorControlSetOutput.vi"("Output"=w315, "MotorControlDevRef"=w320) -> ()  [unwired: 7 in, 3 out]
                    }
                  }
                  frame #1 {
                    w324 = FALSE ("btn_intake level 2")
                    w327 = 0.0 ("Output")
                    n185 = call <vilib>:"WPI_MotorControlSetOutput.vi"("Output"=w327, "MotorControlDevRef"=w326) -> ()  [unwired: 7 in, 3 out]
                    n186 = call <vilib>:"WPI_MotorControlSetOutput.vi"("Output"=w327, "MotorControlDevRef"=w325) -> ()  [unwired: 7 in, 3 out]
                    n187 = global write "Robot Global Data.vi" "btn_intake level 2"(w324) -> ()
                    n188 = global write "Robot Global Data.vi" "btn_intake level 3"(w324) -> ()
                  }
                }
              }
            }
          }
          frame True {
            w329 = 0.35 ("t")
            n189 = global read "Robot Global Data.vi" "btn_intakearm_up (manual)"() -> (w332:bool)
            n190 = global read "Robot Global Data.vi" "btn_intakearm_down (manual)"() -> (w331:bool)
            n191 = Negate(x=w329) -> (-x=w328:dbl)
            n192 = Select(t=w329, s=w332, f=0.0) -> (s? t:f=w334:dbl)
            n193 = Select(t=w328, s=w331, f=w334) -> (s? t:f=w333:dbl)
            n194 = call <vilib>:"WPI_MotorControlSetOutput.vi"("Output"=w333, "MotorControlDevRef"=w336) -> ()  [unwired: 7 in, 3 out]
            n195 = call <vilib>:"WPI_MotorControlSetOutput.vi"("Output"=w333, "MotorControlDevRef"=w335) -> ()  [unwired: 7 in, 3 out]
          }
        }
        n196 = Wait (ms)(milliseconds to wait=u32 10) -> ()  [unwired: 1 out]
      }
    }
    frame Disabled {
    }
  }
  n197 = disable-structure shown="Enabled" {
    frame Disabled {
    }
    frame Enabled {
      # "Shooter 2"
      n198 = call <vilib>:"WPI_MotorControlRefNum Registry Get.vi"("refnum name"="Shooter") -> ("MotorControlDevRef"=w339:T12)  [unwired: 9 in, 1 out]
      n199 = call <vilib>:"WPI_MotorControlRefNum Registry Get.vi"("refnum name"="Intake") -> ("MotorControlDevRef"=w337:T12)  [unwired: 9 in, 1 out]
      n200 = while {
        tunnel: w339 -> [w357]
        tunnel: w337 -> [w348]
        stop <- FALSE stop-if-true
        # "if shooter wheel is off"
        n201 = Wait (ms)(milliseconds to wait=u32 10) -> ()  [unwired: 1 out]
        n202 = global read "Robot Global Data.vi" "Shooter wheel"() -> (w362:bool)
        n203 = call <vilib>:"WPI_CANTalonSRX_SetPID.vi"("CAN Talon SRX Ref"=w357, "P"="P 2", "I"="I 2", "D"="D 2", "F"="F 2", "I Zone"="I Zone 2", "Ramp Rate"="Ramp Rate 2") -> ("CAN Talon SRX Ref"=w346:T12)  [unwired: 7 in, 1 out]
        n204 = call-poly <vilib>:"NT Read Value.vi"("Name"="Shooter") -> ("Numeric"=w360:dbl)  [unwired: 9 in, 1 out]
        n205 = call <vilib>:"WPI_CANTalonSRX_GetStatus.vi"("CAN Talon SRX Ref"=w346) -> ("Talon SRX Status"=w345:T19)  [unwired: 8 in, 2 out]
        n206 = Unbundle By Name(w345) -> ("Sensor Velocity"=w344:dbl)
        "Sensor Velocity" <- w344
        "Motor Output 2" <- w344
        n207 = call-poly <vilib>:"NT Write Value.vi"("Numeric"=w344, "Name"="Shooter Velocity ") -> ()  [unwired: 9 in, 1 out]
        n208 = Multiply(x=w360, y=6.8266667) -> (x*y=w359:dbl)
        n209 = case shown="False" w362 {
          tunnel: w359 -> [_ w386]
          tunnel: w346 -> [w381 w385]
          tunnel: [w380 w384] -> w347
          frame False {
            n210 = call <vilib>:"WPI_CANTalonSRX_ChangeMode.vi"("Output"=0.0, "Control Mode"=WPI_CANTalonSRX_APIControlMode."Speed", "CAN Talon SRX Ref"=w381) -> ("CAN Talon SRX Ref"=w380:T12)  [unwired: 7 in, 1 out]
          }
          frame True {
            # "start running at x rpms"
            n211 = Negate(x=w386) -> (-x=w387:dbl)
            n212 = call <vilib>:"WPI_CANTalonSRX_ChangeMode.vi"("Output"=w387, "Control Mode"=WPI_CANTalonSRX_APIControlMode."Speed", "CAN Talon SRX Ref"=w385) -> ("CAN Talon SRX Ref"=w384:T12)  [unwired: 7 in, 1 out]
          }
        }
        n213 = global read "Robot Global Data.vi" "Shooter wheel"() -> (w350:bool)
        n214 = global read "Robot Global Data.vi" "Loaded?"() -> (w341:bool)
        n215 = global read "Robot Global Data.vi" "Shoot!"() -> (w342:bool)
        n216 = Compound Arithmetic op=AND(w341, w350, w342) -> (w349:bool)
        n217 = case shown="True" w349 {
          tunnel: w348 -> [_ w366]
          tunnel: w347 -> [_ w365]
          frame False {
          }
          frame True {
            n218 = stacked-sequence {
              tunnel: w366 -> [_ w373 _]
              tunnel: w365 -> [_ _ w376]
              frame #0 {
                n219 = global write "Robot Global Data.vi" "Shooting?"(TRUE ("btn_intake level 3")) -> ()
                n220 = Wait (ms)(milliseconds to wait=u32 100) -> ()  [unwired: 1 out]
              }
              frame #1 {
                n221 = call-poly <vilib>:"NT Read Value.vi"("Name"="Shoot outtake speed") -> ("Numeric"=w372:dbl)  [unwired: 9 in, 1 out]
                n222 = call <vilib>:"WPI_MotorControlSetOutput.vi"("Output"=w372, "MotorControlDevRef"=w373) -> ()  [unwired: 7 in, 3 out]
                n223 = call-poly <vilib>:"NT Read Value.vi"("Name"="Shoot outtake duration") -> ("Numeric"=w369:dbl)  [unwired: 9 in, 1 out]
                n224 = Wait (ms)(milliseconds to wait=w369) -> ()  [unwired: 1 out]
              }
              frame #2 {
                n225 = global write "Robot Global Data.vi" "Shooter wheel"(FALSE ("Shooter wheel")) -> ()
                n226 = global write "Robot Global Data.vi" "Shooting?"(FALSE ("Shooter wheel")) -> ()
                n227 = call <vilib>:"WPI_CANTalonSRX_ChangeMode.vi"("Output"=0.0, "Control Mode"=WPI_CANTalonSRX_APIControlMode."Speed", "CAN Talon SRX Ref"=w376) -> ()  [unwired: 7 in, 2 out]
                n228 = Wait (ms)(milliseconds to wait=u32 100) -> ()  [unwired: 1 out]
              }
            }
          }
        }
      }
    }
  }
